vi "XW_Linearise_+_temp_comp.vi"(8 "XW2 voltage":dbl[](array[numeric]) format="%.4f", 9 "Calib const":dbl[](array[numeric]) format="%.4f", 11 "XW1 voltage":dbl[](array[numeric]) format="%.4f") -> (0 "V":dbl[](array[numeric]) format="%.2f", 1 "U":dbl[](array[numeric]) format="%.2f", 2 "U2":dbl[](array[numeric]) format="%.2f", 3 "U1":dbl[](array[numeric]) format="%.2f")   [LabVIEW 2020]
uses:
  <vilib>/Analysis/baseanly.llb/Mean (DBL).vi
  XW calib map/XW_Map_Global.vi
  Globals/Meas_global.vi
  Globals/Dynamic_call_global.ph.vi
  <vilib>/Analysis/NI_AALBase.lvlib
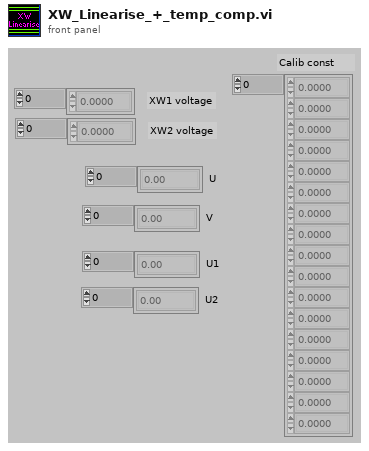
[diagram p1: front panel]
types:
  T1 = cluster{"Calib const[0]":dbl, "Calib const[1]":dbl, "Calib const[2]":dbl, "Calib const[3]":dbl, "Calib const[4]":dbl, "Calib const[5]":dbl, "Calib const[6]":dbl, "Calib const[7]":dbl, "Calib const[8]":dbl, "Calib const[9]":dbl, "Calib const[10]":dbl, "Calib const[11]":dbl, "Calib const[12]":dbl, "Calib const[13]":dbl, "Calib const[14]":dbl, "Calib const[15]":dbl, "Calib const[16]":dbl, "Calib const[17]":dbl}
  T2 = typedef "Map method.ctl" = enum16{"Triangle mesh", "Polynomial surface", "Const. Psi_eff (std.)", "Psi_eff = f(Umagn.)", "Psi_eff, k = f(Umagn.)"}
  T3 = typedef "Trimmed down TreeNode2D.ctl" = cluster{"Xmax":dbl, "Xmin":dbl, "Ymax":dbl, "Ymin":dbl, "Xc":dbl, "Yc":dbl, "ObjIndexList":i32[], "NodeQ1Index":i32, "NodeQ2Index":i32, "NodeQ3Index":i32, "NodeQ4Index":i32}
  T4 = typedef "Triangle2D.ctl" = cluster{"V10":dbl[], "V20":dbl[], "1/det":dbl, "V0":cluster{"PosVector":dbl[], "ValueVector":dbl[]}, "V1":cluster{"PosVector":dbl[], "ValueVector":dbl[]}, "V2":cluster{"PosVector":dbl[], "ValueVector":dbl[]}, "V21":dbl[]}
  T5 = enum16{"2nd component as calculated", "2nd component multipled by -1"}
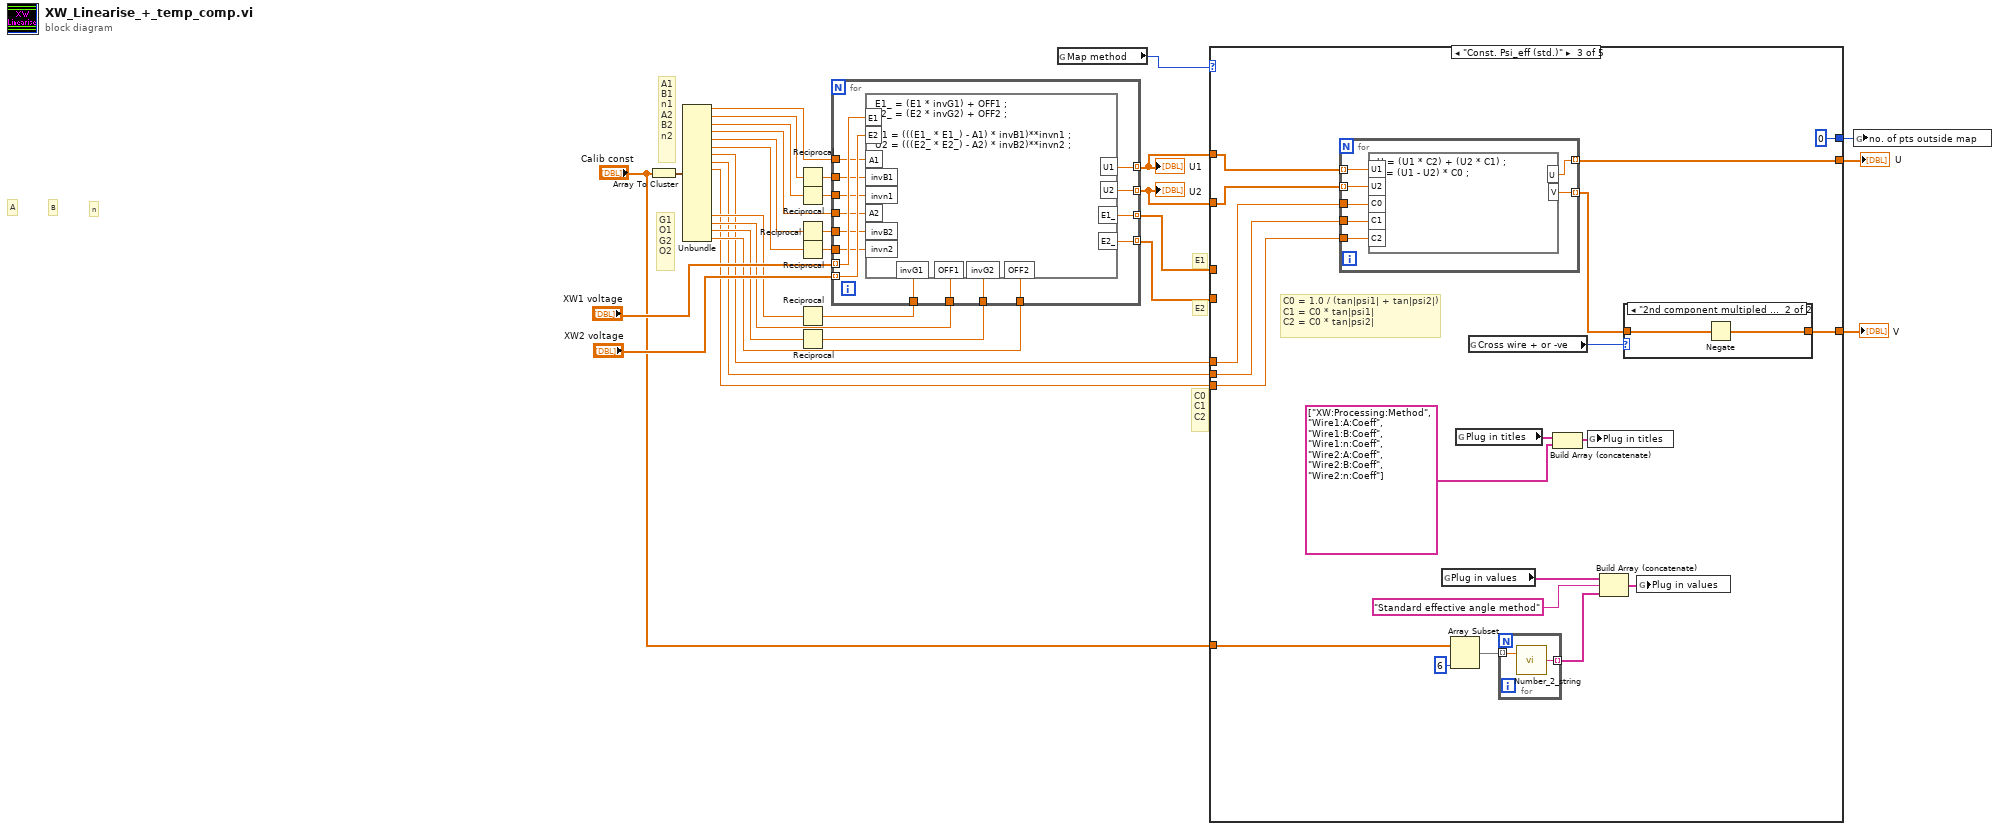
[diagram p0: block diagram]
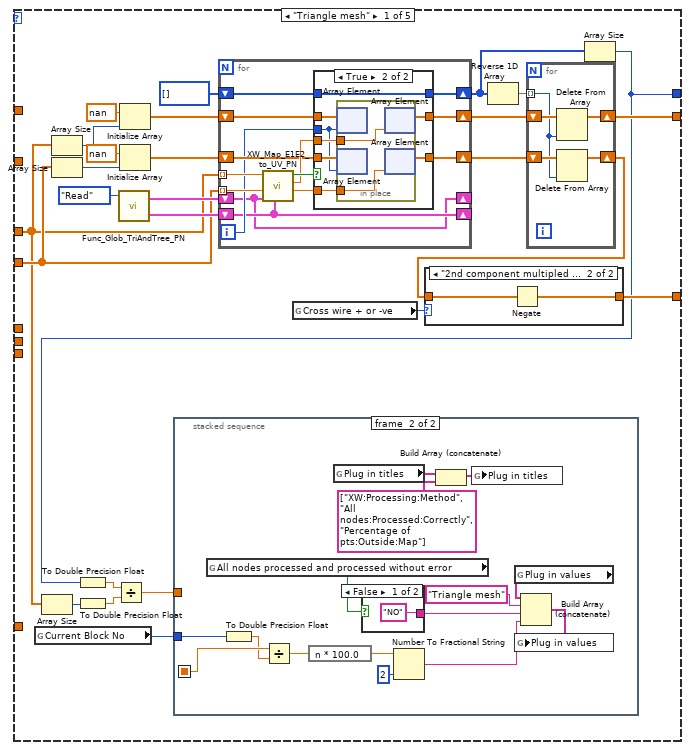
[diagram p2: hidden frame]
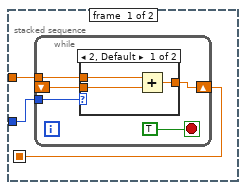
[diagram p3: hidden frame]
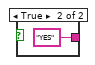
[diagram p5: hidden frame]
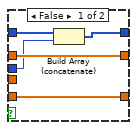
[diagram p6: hidden frame]
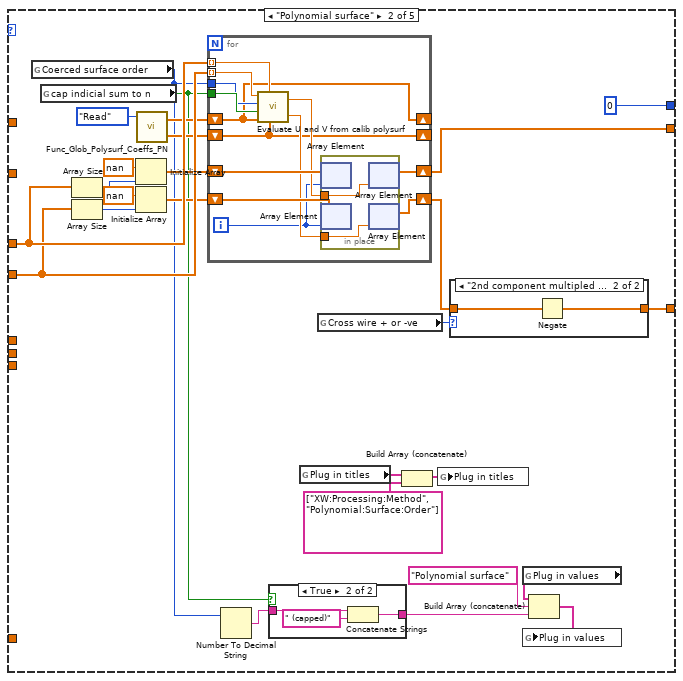
[diagram p8: hidden frame]
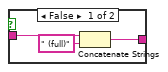
[diagram p9: hidden frame]
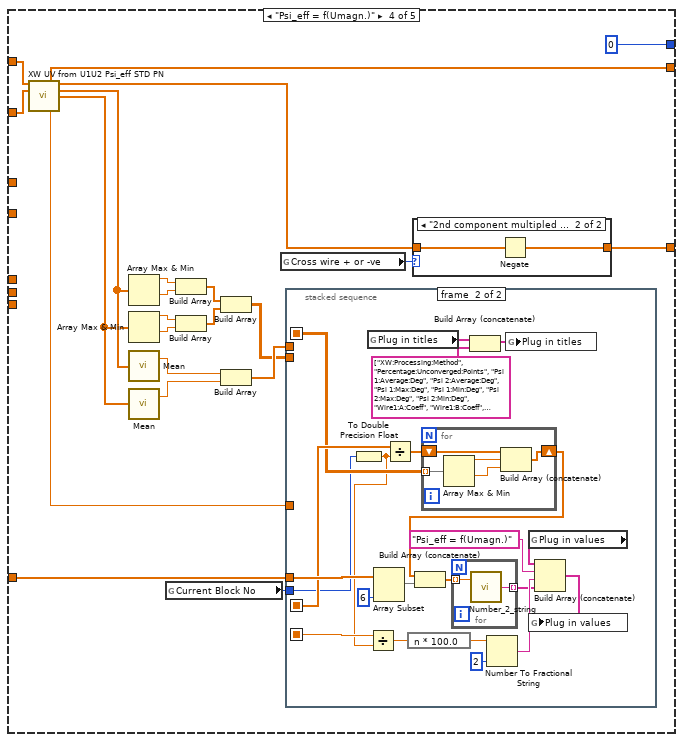
[diagram p12: hidden frame]
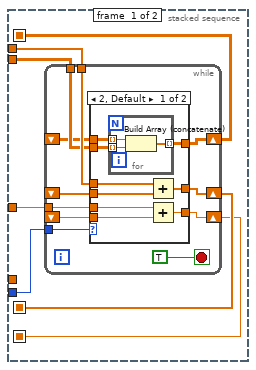
[diagram p13: hidden frame]
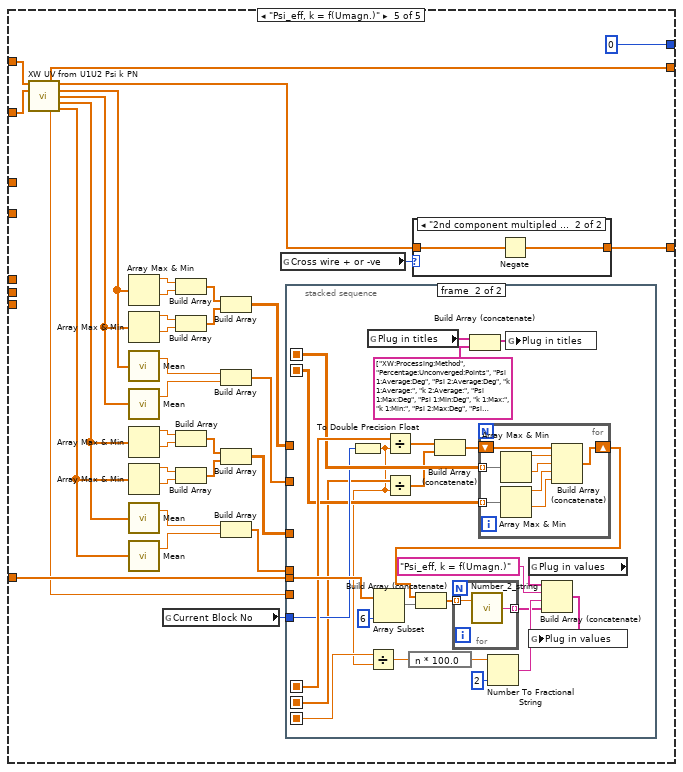
[diagram p16: hidden frame]
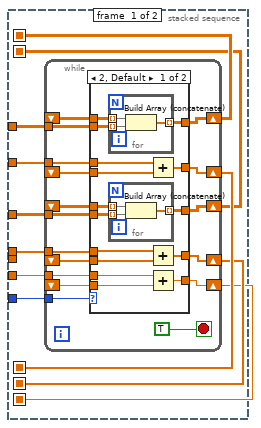
[diagram p17: hidden frame]
diagram:
  # "C0\nC1\nC2"
  # "E2"
  # "E1"
  # "G1\nO1\nG2\nO2"
  # "A1\nB1\nn1\nA2\nB2\nn2"
  # "n"
  # "B"
  # "A"
  n1 = Array To Cluster(array="Calib const") -> (cluster=w31:T1)
  n2 = Unbundle(w31) -> ("Calib const[0]"=w22:dbl, "Calib const[1]"=w16:dbl, "Calib const[2]"=w12:dbl, "Calib const[3]"=w21:dbl, "Calib const[4]"=w14:dbl, "Calib const[5]"=w10:dbl, "Calib const[6]"=w3:dbl, "Calib const[7]"=w2:dbl, "Calib const[8]"=w1:dbl, "Calib const[14]"=w8:dbl, "Calib const[15]"=w19:dbl, "Calib const[16]"=w6:dbl, "Calib const[17]"=w20:dbl)  [unwired: 5 out]
  n3 = Reciprocal(x=w16) -> (1/x=w15:dbl)
  n4 = Reciprocal(x=w12) -> (1/x=w11:dbl)
  n5 = Reciprocal(x=w14) -> (1/x=w13:dbl)
  n6 = Reciprocal(x=w10) -> (1/x=w9:dbl)
  n7 = Reciprocal(x=w8) -> (1/x=w7:dbl)
  n8 = Reciprocal(x=w6) -> (1/x=w5:dbl)
  n9 = for {
    tunnel: [w47] -> w26 mode=indexing
    tunnel: [w46] -> w25 mode=indexing
    tunnel: [w45] -> w18 mode=indexing
    tunnel: [w44] -> w17 mode=indexing
    tunnel: "XW1 voltage" -> [w43] mode=indexing
    tunnel: "XW2 voltage" -> [w42] mode=indexing
    tunnel: w22 -> [w41]
    tunnel: w15 -> [w40]
    tunnel: w11 -> [w39]
    tunnel: w21 -> [w38]
    tunnel: w13 -> [w37]
    tunnel: w9 -> [w36]
    tunnel: w20 -> [w35]
    tunnel: w5 -> [w34]
    tunnel: w19 -> [w33]
    tunnel: w7 -> [w32]
    n10 = formula code="E1_ = (E1 * invG1) + OFF1 ;\nE2_ = (E2 * invG2) + OFF2 ;\n\nU1 = (((E1_ * E1_) - A1) * invB1)**invn1 ;\nU2 = (((E2_ * E2_) - A2) * invB2)**invn2 ;"("E1"=w43, "E2"=w42, "A1"=w41, "invB1"=w40, "invn1"=w39, "A2"=w38, "invB2"=w37, "invn2"=w36, "invG1"=w32, "OFF1"=w33, "invG2"=w34, "OFF2"=w35) -> ("E1_"=w47:dbl, "E2_"=w46:dbl, "U1"=w45:dbl, "U2"=w44:dbl)
  }
  "U2" <- w17
  "U1" <- w18
  n11 = global read "XW_Map_Global.vi" "Map method"() -> (w28:T2)
  n12 = case shown="\"Const. Psi_eff (std.)\"" w28 {
    tunnel: w25 -> [w54 w158 _ _ _]
    tunnel: w26 -> [w50 w159 _ _ _]
    tunnel: [w60 w155 w205 w241 w339] -> w30
    tunnel: [w73 w165 w207 w227 w336] -> w29
    tunnel: [w55 0 0 0 0] -> w27
    tunnel: w18 -> [_ _ w204 w243 w341]
    tunnel: w17 -> [_ _ w203 w242 w340]
    tunnel: "Calib const" -> [_ _ w199 w223 w322]
    tunnel: w3 -> [_ _ w202 _ _]
    tunnel: w2 -> [_ _ w201 _ _]
    tunnel: w1 -> [_ _ w200 _ _]
    frame "Triangle mesh" {
      n13 = global read "Meas_global.vi" "Current Block No"() -> (w49:i32)
      n14 = Array Size(array=w50) -> (size(s)=w53:i32)
      n15 = Array Size(array=w50) -> (size(s)=w69:i32)
      n16 = Array Size(array=w54) -> (size(s)=w68:i32)
      n17 = To Double Precision Float(number=w53) -> (double precision float=w51:dbl)
      n18 = call "Func_Glob_TriAndTree_PN.vi"("Action"=enum16{"Read", "Write"}."Read") -> ("Trimmed down TreeNode array OUT"=w56:T3[], "Corrected triangles OUT"=w57:T4[])  [unwired: 2 in]
      n19 = Initialize Array(nan ("element"), w69) -> (w66:dbl[])
      n20 = Initialize Array(nan ("element"), w68) -> (w67:dbl[])
      n21 = for {
        tunnel: w50 -> [w121] mode=indexing
        tunnel: w54 -> [w120] mode=indexing
        shift-right: [w109] -> w59
        shift-left: i32[] [] -> [w108]
        shift-right: [w116] -> w64
        shift-left: w66 -> [w115]
        shift-right: [w113] -> w63
        shift-left: w67 -> [w114]
        shift-right: [w110] -> _
        shift-left: w57 -> [w110]
        shift-right: [w111] -> _
        shift-left: w56 -> [w111]
        i -> [w112]
        n22 = call "XW_Map_E1E2_to_UV_PN.vi"("Trimmed down TreeNode array"=w111, "Triangulated XW Calib Map Mesh"=w110, "(E2 / G2) + O2 (Volts)"=w120, "(E1 / G1) + O1 (Volts)"=w121) -> ("V (m/s)"=w117:dbl, "U (m/s)"=w118:dbl, "Voltages are inside calibrated region"=w119:bool)  [unwired: 5 out]
        n23 = case shown="True" w119 {
          tunnel: w118 -> [_ w130]
          tunnel: w108 -> [w122 w134]
          tunnel: [w123 w134] -> w109
          tunnel: w117 -> [_ w129]
          tunnel: [w126 w132] -> w116
          tunnel: w115 -> [w126 w133]
          tunnel: w114 -> [w125 w131]
          tunnel: [w125 w128] -> w113
          tunnel: w112 -> [w124 w127]
          frame False {
            n24 = Build Array (concatenate)(w122, w124) -> (w123:i32[])
          }
          frame True {
            n25 = in-place {
              in-place-border: w130 -> [w136]
              in-place-border: w129 -> [w135]
              n26 = in-place-array #1(w133, w127) -> ()  [unwired: 1 out]
              n27 = in-place-array #2(w131, w127) -> ()  [unwired: 1 out]
              n28 = in-place-array #1(w136) -> (w132:dbl[])  [unwired: 1 out]
              n29 = in-place-array #2(w135) -> (w128:dbl[])  [unwired: 1 out]
            }
          }
        }
      }
      n30 = global read "Meas_global.vi" "Cross wire + or -ve"() -> (w72:T5)
      n31 = Reverse 1D Array(array=w59) -> (reversed array=w62:i32[])
      n32 = for {
        shift-right: [w104] -> w60
        shift-left: w64 -> [w107]
        shift-right: [w105] -> w61
        shift-left: w63 -> [w106]
        tunnel: w62 -> [w103] mode=indexing
        n33 = Delete From Array(array=w107, index=w103) -> (array with subset deleted=w104:dbl[])  [unwired: 1 in, 1 out]
        n34 = Delete From Array(array=w106, index=w103) -> (array with subset deleted=w105:dbl[])  [unwired: 1 in, 1 out]
      }
      n35 = case shown="\"2nd component multipled by -1\"" w72 {
        tunnel: [w137 w139] -> w73
        tunnel: w61 -> [w137 w138]
        frame "2nd component as calculated" {
        }
        frame "2nd component multipled by -1" {
          n36 = Negate(x=w138) -> (-x=w139:dbl[])
        }
      }
      n37 = Array Size(array=w59) -> (size(s)=w55:i32)
      n38 = To Double Precision Float(number=w55) -> (double precision float=w52:dbl)
      n39 = Divide(x=w52, y=w51) -> (x/y=w48:dbl)
      n40 = stacked-sequence {
        seq-local: [w76 _] -> [_ w99]
        tunnel: w49 -> [w75 w100]
        tunnel: w48 -> [w74 _]
        frame #0 {
          n41 = while {
            shift-right: [w81] -> w76
            shift-left: _ -> [w78]
            tunnel: w75 -> [w79]
            tunnel: w74 -> [w77]
            stop <- TRUE stop-if-true
            n42 = case shown="2, Default" w79 {
              tunnel: w78 -> [w83 _]
              tunnel: [w84 w85] -> w81
              tunnel: w77 -> [w82 w85]
              frame 2, Default {
                n43 = Add(x=w82, y=w83) -> (x+y=w84:dbl)
              }
              frame 1 {
              }
            }
          }
        }
        frame #1 {
          n44 = global read "XW_Map_Global.vi" "All nodes processed and processed without error"() -> (w95:bool)
          n45 = To Double Precision Float(number=w100) -> (double precision float=w97:dbl)
          n46 = Divide(x=w99, y=w97) -> (x/y=w87:dbl)
          n47 = expression code="n * 100.0"(w87) -> (w86:dbl)
          n48 = global read "Dynamic_call_global.ph.vi" "Plug in titles"() -> (w91:string[])
          n49 = case shown="False" w95 {
            tunnel: ["NO" "YES"] -> w96
            frame False {
            }
            frame True {
            }
          }
          n50 = Number To Fractional String(number=w86, precision (6)=i16 2) -> (F-format string=w88:string)  [unwired: 2 out]
          n51 = Build Array (concatenate)(w91, string[] ["XW:Processing:Method", "All nodes:Processed:Correctly", "Percentage of pts:Outside:Map"] ("array")) -> (w89:string[])
          n52 = global write "Dynamic_call_global.ph.vi" "Plug in titles"(w89) -> ()
          n53 = global read "Dynamic_call_global.ph.vi" "Plug in values"() -> (w93:string[])
          n54 = Build Array (concatenate)(w93, "Triangle mesh", w96, w88) -> (w90:string[])
          n55 = global write "Dynamic_call_global.ph.vi" "Plug in values"(w90) -> ()
        }
      }
    }
    frame "Polynomial surface" {
      n56 = global read "XW_Map_Global.vi" "Coerced surface order"() -> (w149:i32)
      n57 = global read "XW_Map_Global.vi" "cap indicial sum to n"() -> (w148:bool)
      n58 = Array Size(array=w159) -> (size(s)=w161:i32)
      n59 = Array Size(array=w158) -> (size(s)=w160:i32)
      n60 = Initialize Array(nan ("element"), w161) -> (w157:dbl[])
      n61 = Initialize Array(nan ("element"), w160) -> (w156:dbl[])
      n62 = call "Func_Glob_Polysurf_Coeffs_PN.vi"("Action"=enum16{"Read", "Write"}."Read") -> ("alpha(rad) coeffs OUT"=w151:dbl[], "Ucal coeffs OUT"=w152:dbl[])  [unwired: 2 in]
      n63 = for {
        tunnel: w159 -> [w184] mode=indexing
        tunnel: w158 -> [w183] mode=indexing
        tunnel: w148 -> [w182]
        shift-right: [w180] -> w154
        shift-left: w156 -> [w178]
        shift-right: [w181] -> w155
        shift-left: w157 -> [w179]
        tunnel: w149 -> [w174]
        shift-right: [w173] -> _
        shift-left: w151 -> [w173]
        shift-right: [w172] -> _
        shift-left: w152 -> [w172]
        i -> [w175]
        n64 = call "Evaluate U and V from calib polysurf.vi"("alpha(rad) coeffs"=w173, "E1 / G1 + O1"=w184, "Ucal coeffs"=w172, "cap indicial sum to n"=w182, "surface order (n)"=w174, "E2 / G2 + O2"=w183) -> ("V (m/s)"=w177:dbl, "U (m/s)"=w176:dbl)
        n65 = in-place {
          in-place-border: w176 -> [w186]
          in-place-border: w177 -> [w185]
          n66 = in-place-array #3(w179, w175) -> ()  [unwired: 1 out]
          n67 = in-place-array #4(w178, w175) -> ()  [unwired: 1 out]
          n68 = in-place-array #3(w186) -> (w181:dbl[])  [unwired: 1 out]
          n69 = in-place-array #4(w185) -> (w180:dbl[])  [unwired: 1 out]
        }
      }
      n70 = Number To Decimal String(number=w149) -> (decimal integer string=w140:string)  [unwired: 1 out]
      n71 = case shown="True" w148 {
        tunnel: [w166 w169] -> w141
        tunnel: w140 -> [w168 w171]
        frame False {
          n72 = Concatenate Strings(w168, " (full)") -> (w166:string)
        }
        frame True {
          n73 = Concatenate Strings(w171, " (capped)") -> (w169:string)
        }
      }
      n74 = global read "Dynamic_call_global.ph.vi" "Plug in titles"() -> (w145:string[])
      n75 = global read "Meas_global.vi" "Cross wire + or -ve"() -> (w164:T5)
      n76 = Build Array (concatenate)(w145, string[] ["XW:Processing:Method", "Polynomial:Surface:Order"] ("array")) -> (w147:string[])
      n77 = global write "Dynamic_call_global.ph.vi" "Plug in titles"(w147) -> ()
      n78 = case shown="\"2nd component multipled by -1\"" w164 {
        tunnel: [w187 w189] -> w165
        tunnel: w154 -> [w187 w188]
        frame "2nd component as calculated" {
        }
        frame "2nd component multipled by -1" {
          n79 = Negate(x=w188) -> (-x=w189:dbl[])
        }
      }
      n80 = global read "Dynamic_call_global.ph.vi" "Plug in values"() -> (w143:string[])
      n81 = Build Array (concatenate)(w143, "Polynomial surface", w141) -> (w146:string[])
      n82 = global write "Dynamic_call_global.ph.vi" "Plug in values"(w146) -> ()
    }
    frame "Const. Psi_eff (std.)" {
      # "C0 = 1.0 / (tan|psi1| + tan|psi2|)\nC1 = C0 * tan|psi1|\nC2 = C0 * tan|psi2|"
      n83 = for {
        tunnel: [w218] -> w206 mode=indexing
        tunnel: [w217] -> w205 mode=indexing
        tunnel: w204 -> [w216] mode=indexing
        tunnel: w203 -> [w215] mode=indexing
        tunnel: w202 -> [w214]
        tunnel: w201 -> [w213]
        tunnel: w200 -> [w212]
        n84 = formula code="U = (U1 * C2) + (U2 * C1) ;\nV = (U1 - U2) * C0 ;"("U1"=w216, "U2"=w215, "C1"=w213, "C2"=w212, "C0"=w214) -> ("U"=w217:dbl, "V"=w218:dbl)
      }
      n85 = global read "Dynamic_call_global.ph.vi" "Plug in values"() -> (w191:string[])
      n86 = Array Subset(array=w199, length=6) -> (w192:dbl[])  [unwired: 1 in]
      n87 = global read "Dynamic_call_global.ph.vi" "Plug in titles"() -> (w196:string[])
      n88 = global read "Meas_global.vi" "Cross wire + or -ve"() -> (w208:T5)
      n89 = for {
        tunnel: w192 -> [w211] mode=indexing
        tunnel: [w210] -> w195 mode=indexing
        n90 = call "Number_2_string.vi"("number"=w211) -> ("String"=w210:string)  [unwired: 1 in]
      }
      n91 = Build Array (concatenate)(w196, string[] ["XW:Processing:Method", "Wire1:A:Coeff", "Wire1:B:Coeff", "Wire1:n:Coeff", "Wire2:A:Coeff", "Wire2:B:Coeff", "Wire2:n:Coeff"] ("array")) -> (w198:string[])
      n92 = global write "Dynamic_call_global.ph.vi" "Plug in titles"(w198) -> ()
      n93 = Build Array (concatenate)(w191, "Standard effective angle method", w195) -> (w197:string[])
      n94 = case shown="\"2nd component multipled by -1\"" w208 {
        tunnel: [w219 w221] -> w207
        tunnel: w206 -> [w219 w220]
        frame "2nd component as calculated" {
        }
        frame "2nd component multipled by -1" {
          n95 = Negate(x=w220) -> (-x=w221:dbl[])
        }
      }
      n96 = global write "Dynamic_call_global.ph.vi" "Plug in values"(w197) -> ()
    }
    frame "Psi_eff = f(Umagn.)" {
      n97 = call "XW UV from U1U2 Psi_eff STD PN.vi"("U1cal (m/s)"=w243, "U2cal (m/s)"=w242) -> ("U (m/s)"=w241:dbl[], "V (m/s)"=w228:dbl[], "Psi1 (deg)"=w239:dbl[], "Psi2 (deg)"=w238:dbl[], "Unconverged points (fraction)"=w222:dbl)  [unwired: 9 out]
      n98 = Array Max & Min(array=w239) -> (max value=w234:dbl, min value=w235:dbl)  [unwired: 2 out]
      n99 = Array Max & Min(array=w238) -> (max value=w233:dbl, min value=w232:dbl)  [unwired: 2 out]
      n100 = call-poly <vilib>:"Mean.vi"("X"=w239) -> ("mean"=w237:dbl)  [unwired: 1 out]
      n101 = call-poly <vilib>:"Mean.vi"("X"=w238) -> ("mean"=w236:dbl)  [unwired: 1 out]
      n102 = global read "Meas_global.vi" "Current Block No"() -> (w226:i32)
      n103 = Build Array(w234, w235) -> (w230:dbl[])
      n104 = Build Array(w233, w232) -> (w231:dbl[])
      n105 = Build Array(w230, w231) -> (w224:dbl[][])
      n106 = Build Array(w237, w236) -> (w225:dbl[])
      n107 = global read "Meas_global.vi" "Cross wire + or -ve"() -> (w229:T5)
      n108 = stacked-sequence {
        seq-local: [w248 _] -> [_ w297]
        seq-local: [w247 _] -> [_ w296]
        seq-local: [w244 _] -> [_ w294]
        tunnel: w225 -> [w250 _]
        tunnel: w224 -> [w249 _]
        tunnel: w223 -> [_ w298]
        tunnel: w226 -> [w246 w295]
        tunnel: w222 -> [w245 _]
        frame #0 {
          n109 = while {
            shift-right: [w259] -> w248
            shift-left: _ -> [w260]
            tunnel: w250 -> [w261]
            shift-right: [w257] -> w247
            shift-left: _ -> [w255]
            tunnel: w249 -> [w256]
            tunnel: w246 -> [w254]
            shift-right: [w251] -> w244
            shift-left: _ -> [w253]
            tunnel: w245 -> [w252]
            stop <- TRUE stop-if-true
            n110 = case shown="2, Default" w254 {
              tunnel: w261 -> [w270 w276]
              tunnel: w260 -> [w269 _]
              tunnel: [w268 w276] -> w259
              tunnel: [w265 w275] -> w257
              tunnel: w256 -> [w266 w275]
              tunnel: w255 -> [w267 _]
              tunnel: [w264 w274] -> w251
              tunnel: w253 -> [w263 _]
              tunnel: w252 -> [w262 w274]
              frame 2, Default {
                n111 = for {
                  tunnel: w267 -> [w273] mode=indexing
                  tunnel: w266 -> [w272] mode=indexing
                  tunnel: [w271] -> w265 mode=indexing
                  n112 = Build Array (concatenate)(w273, w272) -> (w271:dbl[])
                }
                n113 = Add(x=w270, y=w269) -> (x+y=w268:dbl[])
                n114 = Add(x=w262, y=w263) -> (x+y=w264:dbl)
              }
              frame 1 {
              }
            }
          }
        }
        frame #1 {
          n115 = To Double Precision Float(number=w295) -> (double precision float=w279:dbl)
          n116 = global read "Dynamic_call_global.ph.vi" "Plug in titles"() -> (w291:string[])
          n117 = Divide(x=w294, y=w279) -> (x/y=w278:dbl)
          n118 = Array Subset(array=w298, length=6) -> (w288:dbl[])  [unwired: 1 in]
          n119 = Divide(x=w297, y=w279) -> (x/y=w286:dbl[])
          n120 = expression code="n * 100.0"(w278) -> (w277:dbl)
          n121 = for {
            tunnel: w296 -> [w303] mode=indexing
            shift-right: [w299] -> w285
            shift-left: w286 -> [w302]
            n122 = Array Max & Min(array=w303) -> (max value=w301:dbl, min value=w300:dbl)  [unwired: 2 out]
            n123 = Build Array (concatenate)(w302, w301, w300) -> (w299:dbl[])
          }
          n124 = Build Array (concatenate)(w285, w288) -> (w287:dbl[])
          n125 = for {
            tunnel: w287 -> [w305] mode=indexing
            tunnel: [w304] -> w280 mode=indexing
            n126 = call "Number_2_string.vi"("number"=w305) -> ("String"=w304:string)  [unwired: 1 in]
          }
          n127 = Build Array (concatenate)(w291, string[] ["XW:Processing:Method", "Percentage:Unconverged:Points", "Psi 1:Average:Deg", "Psi 2:Average:Deg", "Psi 1:Max:Deg", "Psi 1:Min:Deg", "Psi 2:Max:Deg", "Psi 2:Min:Deg", "Wire1:A:Coeff", "Wire1:B:Coeff", "Wire1:n:Coeff", "Wire2:A:Coeff", "Wire2:B:Coeff", "Wire2:n:Coeff"] ("array")) -> (w293:string[])
          n128 = Number To Fractional String(number=w277, precision (6)=i16 2) -> (F-format string=w281:string)  [unwired: 2 out]
          n129 = global write "Dynamic_call_global.ph.vi" "Plug in titles"(w293) -> ()
          n130 = global read "Dynamic_call_global.ph.vi" "Plug in values"() -> (w284:string[])
          n131 = Build Array (concatenate)(w284, "Psi_eff = f(Umagn.)", w281, w280) -> (w292:string[])
          n132 = global write "Dynamic_call_global.ph.vi" "Plug in values"(w292) -> ()
        }
      }
      n133 = case shown="\"2nd component multipled by -1\"" w229 {
        tunnel: [w306 w308] -> w227
        tunnel: w228 -> [w306 w307]
        frame "2nd component as calculated" {
        }
        frame "2nd component multipled by -1" {
          n134 = Negate(x=w307) -> (-x=w308:dbl[])
        }
      }
    }
    frame "Psi_eff, k = f(Umagn.)" {
      n135 = call "XW UV from U1U2 Psi k PN.vi"("U1cal (m/s)"=w341, "U2cal (m/s)"=w340) -> ("U (m/s)"=w339:dbl[], "V (m/s)"=w337:dbl[], "Psi1 (deg)"=w327:dbl[], "Psi2 (deg)"=w326:dbl[], "k1"=w313:dbl[], "Unconverged points (fraction)"=w309:dbl, "k2"=w312:dbl[])  [unwired: 7 out]
      n136 = Array Max & Min(array=w327) -> (max value=w332:dbl, min value=w333:dbl)  [unwired: 2 out]
      n137 = Array Max & Min(array=w326) -> (max value=w331:dbl, min value=w330:dbl)  [unwired: 2 out]
      n138 = call-poly <vilib>:"Mean.vi"("X"=w327) -> ("mean"=w335:dbl)  [unwired: 1 out]
      n139 = call-poly <vilib>:"Mean.vi"("X"=w326) -> ("mean"=w334:dbl)  [unwired: 1 out]
      n140 = Array Max & Min(array=w313) -> (max value=w317:dbl, min value=w316:dbl)  [unwired: 2 out]
      n141 = Array Max & Min(array=w312) -> (max value=w318:dbl, min value=w319:dbl)  [unwired: 2 out]
      n142 = call-poly <vilib>:"Mean.vi"("X"=w313) -> ("mean"=w314:dbl)  [unwired: 1 out]
      n143 = call-poly <vilib>:"Mean.vi"("X"=w312) -> ("mean"=w315:dbl)  [unwired: 1 out]
      n144 = global read "Meas_global.vi" "Current Block No"() -> (w323:i32)
      n145 = Build Array(w332, w333) -> (w328:dbl[])
      n146 = Build Array(w331, w330) -> (w329:dbl[])
      n147 = Build Array(w317, w316) -> (w321:dbl[])
      n148 = Build Array(w318, w319) -> (w320:dbl[])
      n149 = Build Array(w328, w329) -> (w325:dbl[][])
      n150 = Build Array(w335, w334) -> (w324:dbl[])
      n151 = Build Array(w321, w320) -> (w310:dbl[][])
      n152 = Build Array(w314, w315) -> (w311:dbl[])
      n153 = global read "Meas_global.vi" "Cross wire + or -ve"() -> (w338:T5)
      n154 = stacked-sequence {
        seq-local: [w351 _] -> [_ w421]
        seq-local: [w350 _] -> [_ w420]
        seq-local: [w346 _] -> [_ w418]
        seq-local: [w345 _] -> [_ w417]
        seq-local: [w343 _] -> [_ w416]
        tunnel: w324 -> [w353 _]
        tunnel: w325 -> [w352 _]
        tunnel: w322 -> [_ w422]
        tunnel: w323 -> [w349 w419]
        tunnel: w311 -> [w348 _]
        tunnel: w310 -> [w347 _]
        tunnel: w309 -> [w344 _]
        frame #0 {
          n155 = while {
            shift-right: [w368] -> w351
            shift-left: _ -> [w369]
            tunnel: w353 -> [w370]
            shift-right: [w366] -> w350
            shift-left: _ -> [w364]
            tunnel: w352 -> [w365]
            tunnel: w349 -> [w363]
            tunnel: w348 -> [w362]
            shift-right: [w360] -> w345
            shift-left: _ -> [w361]
            shift-right: [w359] -> w346
            shift-left: _ -> [w358]
            tunnel: w347 -> [w357]
            tunnel: w344 -> [w356]
            shift-right: [w354] -> w343
            shift-left: _ -> [w355]
            stop <- TRUE stop-if-true
            n156 = case shown="2, Default" w363 {
              tunnel: w370 -> [w385 w396]
              tunnel: w369 -> [w380 _]
              tunnel: [w384 w396] -> w368
              tunnel: [w381 w395] -> w366
              tunnel: w365 -> [w382 w395]
              tunnel: w364 -> [w383 _]
              tunnel: w362 -> [w379 w393]
              tunnel: w361 -> [w378 _]
              tunnel: [w377 w393] -> w360
              tunnel: [w376 w394] -> w359
              tunnel: w358 -> [w375 _]
              tunnel: w357 -> [w374 w394]
              tunnel: w356 -> [w373 w392]
              tunnel: [w372 w392] -> w354
              tunnel: w355 -> [w371 _]
              frame 2, Default {
                n157 = for {
                  tunnel: w383 -> [w391] mode=indexing
                  tunnel: w382 -> [w390] mode=indexing
                  tunnel: [w389] -> w381 mode=indexing
                  n158 = Build Array (concatenate)(w391, w390) -> (w389:dbl[])
                }
                n159 = for {
                  tunnel: w375 -> [w386] mode=indexing
                  tunnel: w374 -> [w388] mode=indexing
                  tunnel: [w387] -> w376 mode=indexing
                  n160 = Build Array (concatenate)(w386, w388) -> (w387:dbl[])
                }
                n161 = Add(x=w385, y=w380) -> (x+y=w384:dbl[])
                n162 = Add(x=w379, y=w378) -> (x+y=w377:dbl[])
                n163 = Add(x=w373, y=w371) -> (x+y=w372:dbl)
              }
              frame 1 {
              }
            }
          }
        }
        frame #1 {
          n164 = To Double Precision Float(number=w419) -> (double precision float=w399:dbl)
          n165 = global read "Dynamic_call_global.ph.vi" "Plug in titles"() -> (w413:string[])
          n166 = Divide(x=w416, y=w399) -> (x/y=w398:dbl)
          n167 = Array Subset(array=w422, length=6) -> (w411:dbl[])  [unwired: 1 in]
          n168 = Divide(x=w421, y=w399) -> (x/y=w409:dbl[])
          n169 = Divide(x=w417, y=w399) -> (x/y=w408:dbl[])
          n170 = expression code="n * 100.0"(w398) -> (w397:dbl)
          n171 = Build Array (concatenate)(w409, w408) -> (w407:dbl[])
          n172 = Build Array (concatenate)(w413, string[] ["XW:Processing:Method", "Percentage:Unconverged:Points", "Psi 1:Average:Deg", "Psi 2:Average:Deg", "k 1:Average:", "k 2:Average:", "Psi 1:Max:Deg", "Psi 1:Min:Deg", "k 1:Max:", "k 1:Min:", "Psi 2:Max:Deg", "Psi 2:Min:Deg", "k 2:Max:", "k 2:Min:", "Wire1:A:Coeff", "Wire1:B:Coeff", "Wire1:n:Coeff", "Wire2:A:Coeff", "Wire2:B:Coeff", "Wire2:n:Coeff"] ("array")) -> (w415:string[])
          n173 = for {
            tunnel: w420 -> [w430] mode=indexing
            shift-right: [w426] -> w403
            shift-left: w407 -> [w429]
            tunnel: w418 -> [w423] mode=indexing
            n174 = Array Max & Min(array=w430) -> (max value=w428:dbl, min value=w427:dbl)  [unwired: 2 out]
            n175 = Array Max & Min(array=w423) -> (max value=w424:dbl, min value=w425:dbl)  [unwired: 2 out]
            n176 = Build Array (concatenate)(w429, w428, w427, w424, w425) -> (w426:dbl[])
          }
          n177 = Build Array (concatenate)(w403, w411) -> (w410:dbl[])
          n178 = for {
            tunnel: w410 -> [w432] mode=indexing
            tunnel: [w431] -> w401 mode=indexing
            n179 = call "Number_2_string.vi"("number"=w432) -> ("String"=w431:string)  [unwired: 1 in]
          }
          n180 = Number To Fractional String(number=w397, precision (6)=i16 2) -> (F-format string=w402:string)  [unwired: 2 out]
          n181 = global write "Dynamic_call_global.ph.vi" "Plug in titles"(w415) -> ()
          n182 = global read "Dynamic_call_global.ph.vi" "Plug in values"() -> (w405:string[])
          n183 = Build Array (concatenate)(w405, "Psi_eff, k = f(Umagn.)", w402, w401) -> (w414:string[])
          n184 = global write "Dynamic_call_global.ph.vi" "Plug in values"(w414) -> ()
        }
      }
      n185 = case shown="\"2nd component multipled by -1\"" w338 {
        tunnel: [w433 w435] -> w336
        tunnel: w337 -> [w433 w434]
        frame "2nd component as calculated" {
        }
        frame "2nd component multipled by -1" {
          n186 = Negate(x=w434) -> (-x=w435:dbl[])
        }
      }
    }
  }
  "U" <- w30
  "V" <- w29
  n187 = global write "XW_Map_Global.vi" "no. of pts outside map"(w27) -> ()
